vi "Read clock rate.vi"(8 "error in (no error)":errorcluster, 11 "build_waveform in":refnum<class "build_waveform.lvclass">) -> (0 "error out":errorcluster, 2 "clock rate":dbl=1200000000.0, 3 "build_waveform out":refnum<class "build_waveform.lvclass">)   [LabVIEW 2019, in "build_waveform.lvclass"]
uses:
  build_waveform.lvclass
  build_waveform.lvclass/build_waveform.ctl
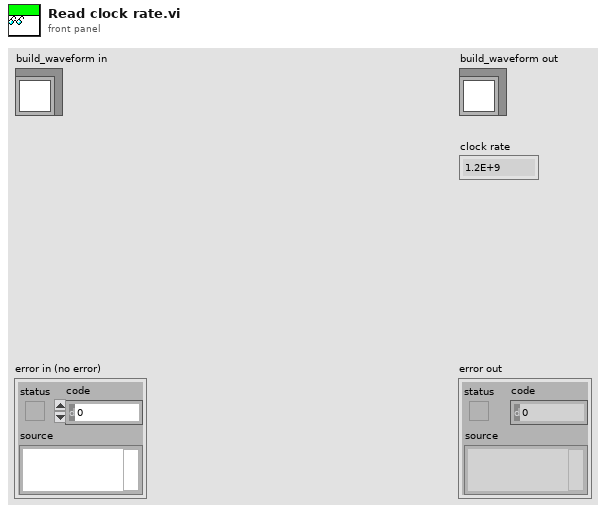
[diagram p1: front panel]
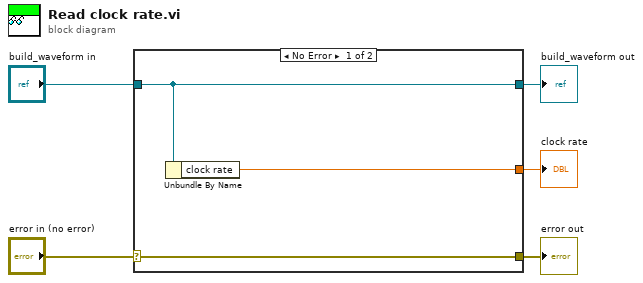
[diagram p0: block diagram]
diagram:
  n1 = case shown="No Error" "error in (no error)" {
    selector: "error in (no error)" -> [w8 w9]
    tunnel: [w8 w9] -> w4
    tunnel: [w7 w10] -> w2
    tunnel: "build_waveform in" -> [w7 w10]
    tunnel: [w6 _] -> w1
    frame No Error {
      n2 = Unbundle By Name(w7) -> ("clock rate"=w6:dbl)
    }
    frame Error {
    }
  }
  "error out" <- w4
  "build_waveform out" <- w2
  "clock rate" <- w1
